vi "Close Dialog.vi"(8 "error in (no error)":errorcluster, 11 "DataGrid Config Dialog in":refnum<class "DataGrid Config Dialog.lvclass">) -> (0 "error out":errorcluster, 3 "DataGrid Config Dialog out":refnum<class "DataGrid Config Dialog.lvclass">)   [LabVIEW 2018, in "DataGrid Config Dialog.lvclass"]
uses:
  DataGrid Config Dialog.lvclass
  DataGrid Config Dialog.lvclass/DataGrid Config Dialog.ctl
  <vilib>/MGI/Panel Manager/Panel/Panel/Panel.lvclass
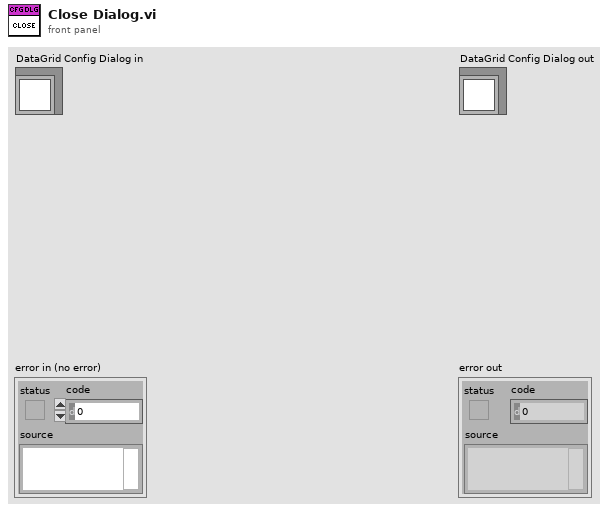
[diagram p1: front panel]
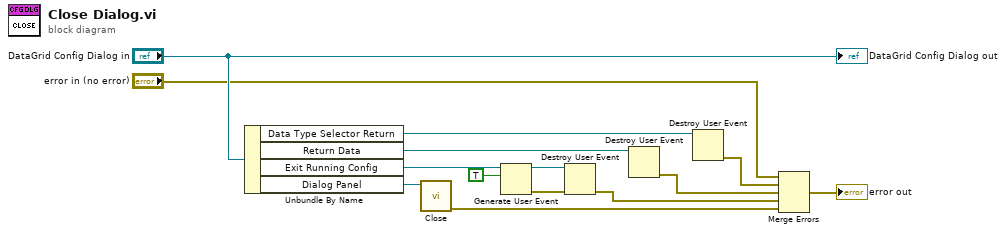
[diagram p0: block diagram]
diagram:
  n1 = Unbundle By Name("DataGrid Config Dialog in") -> ("Data Type Selector Return"=w3:refnum<user-event>, "Return Data"=w4:refnum<user-event>, "Exit Running Config"=w11:refnum<user-event>, "Dialog Panel"=w12:refnum<class "Panel.lvclass">)
  n2 = call-dynamic "Close.vi"("Panel In"=w12) -> ("Error Out"=w8:errorcluster)  [unwired: 10 in]
  n3 = Generate User Event(user event=w11, event data cluster=TRUE ("event data")) -> (user event out=w9:refnum<user-event>, error out=w7:errorcluster)  [unwired: 2 in]
  n4 = Destroy User Event(user event=w9, error in=w7) -> (error out=w6:errorcluster)
  n5 = Destroy User Event(user event=w4) -> (error out=w2:errorcluster)  [unwired: 1 in]
  n6 = Destroy User Event(user event=w3) -> (error out=w1:errorcluster)  [unwired: 1 in]
  n7 = Merge Errors("error in (no error)", w1, w2, w6, w8) -> (→"error out":errorcluster)
  "DataGrid Config Dialog out" <- "DataGrid Config Dialog in"
